vi "Calculate Time Entry.vi"(7 "Recalculate Override (F)":bool, 8 "error in (no error)":errorcluster, 11 "Time Entries in":refnum<class "Time Entries.lvclass">) -> (0 "error out":errorcluster, 2 "Initial Display":string[](array[string]), 3 "Time Entries out":refnum<class "Time Entries.lvclass">)   [LabVIEW 2020, in "Time Entries.lvclass"]
doc: "If the task is still running (i.e. no stop time has been set) then the elapsed time is calculated and the new entry is entered into the display array and the array is available for outputing into the MCLB.\n\n03/2025 Erich Schlieper"
uses:
  Time Entries.lvclass
  Time Entries.lvclass/Time Entries.ctl
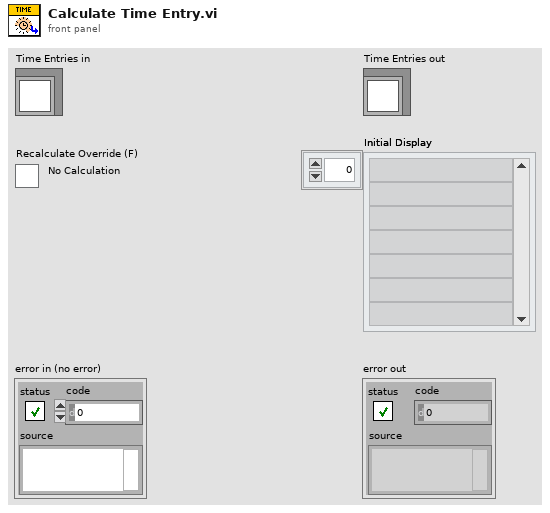
[diagram p1: front panel]
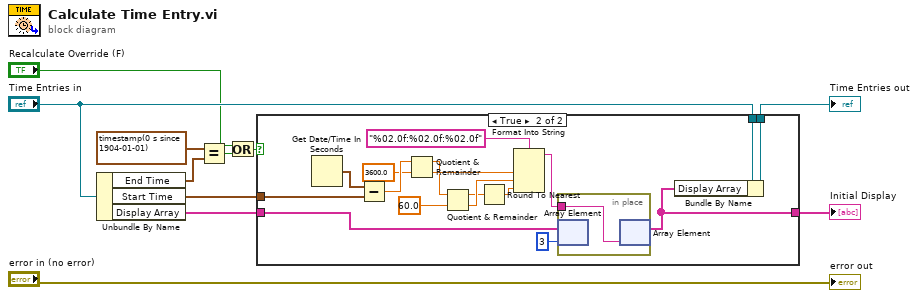
[diagram p0: block diagram]
diagram:
  n1 = Unbundle By Name("Time Entries in") -> ("End Time"=w6:timestamp, "Start Time"=w10:timestamp, "Display Array"=w8:string[])
  n2 = Equal?(x=timestamp(0 s since 1904-01-01) ("End Time"), y=w6) -> (x = y?=w4:bool)
  n3 = Or(x="Recalculate Override (F)", y=w4) -> (x .or. y?=w3:bool)
  n4 = case shown="True" w3 {
    tunnel: "Time Entries in" -> [w12 w30]
    tunnel: w10 -> [_ w28]
    tunnel: [w12 w27] -> w9
    tunnel: w8 -> [w13 w26]
    tunnel: [w13 w24] -> w7
    frame False {
      # "The time entry is comlete and does not need to be recalculated."
    }
    frame True {
      n5 = Get Date/Time In Seconds() -> (seconds since 1Jan1904=w29:timestamp)
      n6 = Subtract(x=w29, y=w28) -> (x-y=w21:dbl)
      n7 = Quotient & Remainder(x=w21, y=3600.0) -> (x-y*floor(x/y)=w14:dbl, floor(x/y)=w20:dbl)
      n8 = Quotient & Remainder(x=w14, y=60.0) -> (x-y*floor(x/y)=w17:dbl, floor(x/y)=w18:dbl)
      n9 = Round To Nearest(number=w17) -> (nearest integer value=w16:dbl)
      n10 = Format Into String(format string="%02.0f:%02.0f:%02.0f" ("time format string (%c)"), w20, w18, w16) -> (resulting string=w23:string)  [unwired: 2 in, 1 out]
      n11 = in-place {
        in-place-border: w23 -> [w31]
        n12 = in-place-array #1(w26, 3) -> ()  [unwired: 1 out]
        n13 = in-place-array #1(w31) -> (w24:string[])  [unwired: 1 out]
      }
      n14 = Bundle By Name(cluster=w30, "Display Array"=w24) -> (w27:refnum<class "Time Entries.lvclass">)
    }
  }
  "Time Entries out" <- w9
  "Initial Display" <- w7
  "error out" <- "error in (no error)"
